vi "PH_4_Pos_Selector.PC set wanted define selector position.vi"(0 "VI in":refnum<vi>, 2 "Wanted Define Selector Position":string, 5 "error in (no error)":errorcluster) -> (14 "VI out":refnum<vi>, 19 "error out":errorcluster)   [LabVIEW 2014, in "PH_4_Pos_Selector.lvlib"]
uses:
  PH_4_Pos_Selector.lvlib
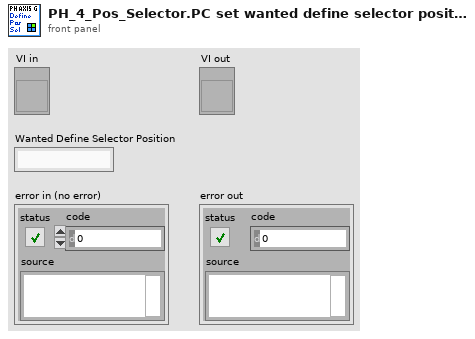
[diagram p1: front panel]
types:
  T1 = typedef "PH_4_Pos_Selector.lvlib/PH_4_Pos_Selector.i attribute.ctl" = cluster{"GUI Refs":cluster{"Position I":refnum<vi>, "Position II":refnum<vi>, "Position III":refnum<vi>, "Position IV":refnum<vi>, "rel. Mode?":refnum<vi>, "Define Selector":refnum<vi>}, "Current Position":T2, "Service ID Position":i32, "Position Array":T3[], "Description Array":string[], "relative Mode":bool, "Wanted Define Selector Position":string}
  T2 = typedef "PH_4_Pos_Selector.lvlib/PH_4_Pos_Selector.Position Selector.ctl" = u16
  T3 = typedef "PH_4_Pos_Selector.lvlib/PH_4_Pos_Selector.Position.ctl" = cluster{"Axis 1":dbl, "Axis 2":dbl}
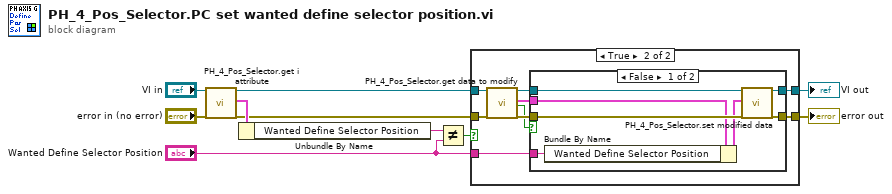
[diagram p0: block diagram]
diagram:
  n1 = call "PH_4_Pos_Selector.get i attribute.vi"("i ref in"="VI in", "error in (no error)"="error in (no error)") -> ("i ref out"=w4:refnum<vi>, "i attribute"=w7:T1, "error out"=w6:errorcluster)  [unwired: 15 in]
  n2 = Unbundle By Name(w7) -> ("Wanted Define Selector Position"=w8:string)
  n3 = Not Equal?(x=w8, y="Wanted Define Selector Position") -> (x != y?=w10:bool)
  n4 = case shown="True" w10 {
    tunnel: [w12 w20] -> w1
    tunnel: [w11 w18] -> w2
    tunnel: w4 -> [w12 w15]
    tunnel: w6 -> [w11 w14]
    tunnel: "Wanted Define Selector Position" -> [_ w13]
    frame False {
    }
    frame True {
      n5 = call "PH_4_Pos_Selector.get data to modify.vi"("i ref in"=w15, "error in (no error)"=w14) -> ("i ref out"=w21:refnum<vi>, "i attribute"=w17:T1, "timed out"=w16:bool, "error out"=w19:errorcluster)  [unwired: 14 in]
      n6 = case shown="False" w16 {
        tunnel: w21 -> [w28 w30]
        tunnel: [w27 w30] -> w20
        tunnel: w19 -> [w26 w29]
        tunnel: [w25 w29] -> w18
        tunnel: w17 -> [w24 _]
        tunnel: w13 -> [w22 _]
        frame False {
          n7 = Bundle By Name(cluster=w24, "Wanted Define Selector Position"=w22) -> (w23:T1)
          n8 = call "PH_4_Pos_Selector.set modified data.vi"("i ref in"=w28, "i attribute"=w23, "error in (no error)"=w26) -> ("i ref out"=w27:refnum<vi>, "error out"=w25:errorcluster)  [unwired: 15 in]
        }
        frame True {
        }
      }
    }
  }
  "error out" <- w2
  "VI out" <- w1
